vi "ST Send.vi"(3 "error in (no error)":errorcluster, 4 "String":string, 5 "VISA resource name":refnum<visa-resource-name>) -> (0 "error out":errorcluster, 1 "return count":u32, 2 "VISA resource name out":refnum<visa-resource-name>)   [LabVIEW 2009]
doc: "This VI sends a character string to the ST Robotic R17 after appending a carriage return, \\r."
uses:
  <vilib>/Instr/_visa.llb/VISA Flush IO Buffer Mask.ctl
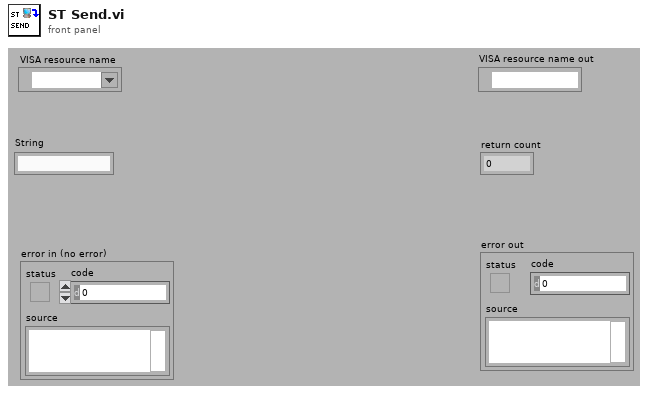
[diagram p1: front panel]
types:
  T1 = typedef "VISA Flush IO Buffer Mask.ctl" = u16
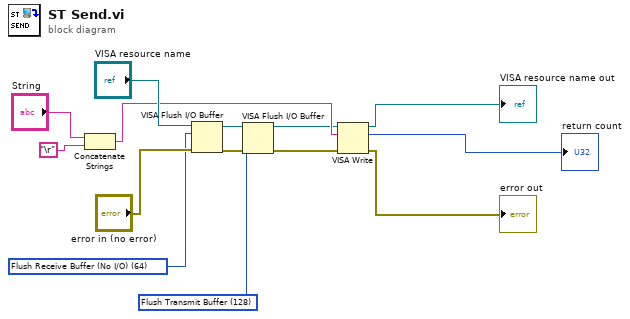
[diagram p0: block diagram]
diagram:
  w1 = T1 128 items=["Flush Receive Buffer"=16, "Write Transmit Buffer to Device"=32, "Flush Receive Buffer (No I/O)"=64, "Flush Transmit Buffer"=128] ("Mask")
  w7 = T1 64 items=["Flush Receive Buffer"=16, "Write Transmit Buffer to Device"=32, "Flush Receive Buffer (No I/O)"=64, "Flush Transmit Buffer"=128] ("Mask")
  n1 = Concatenate Strings("String", "\r") -> (w6:string)
  n2 = VISA Flush I/O Buffer(VISA resource name="VISA resource name", mask (16)=w7, error in (no error)="error in (no error)") -> (VISA resource name out=w2:refnum<visa-resource-name>, error out=w3:errorcluster)
  n3 = VISA Flush I/O Buffer(VISA resource name=w2, mask (16)=w1, error in (no error)=w3) -> (VISA resource name out=w5:refnum<visa-resource-name>, error out=w4:errorcluster)
  n4 = VISA Write(VISA resource name=w5, write buffer=w6, error in (no error)=w4) -> (VISA resource name out=→"VISA resource name out":refnum<visa-resource-name>, return count=→"return count":u32, error out=→"error out":errorcluster)
